vi "CfgLimitLines.vi"(0 "VISA IN":refnum<visa-resource-name>, 1 "Stimulus Start":dbl=1000000000.0, 2 "Stimulus Stop":dbl=2000000000.0, 3 "Amplitude Start":i32=-13, 4 "Amplitude Stop":i32=-14, 5 "Segment Limit":string(combo)="LMAX", 6 "Filename":string="CH1_S11_1", 7 "error in":errorcluster, 8 "Display Limit\n Segments ON/OFF":bool=TRUE, 9 "Channel":i32=1, 10 "Sound ON/OFF":bool=TRUE, 11 "Window":i32=1, 12 "Limit Testing ON/OFF":bool=TRUE, 13 "Segment number":i32=1, 14 "Show Table?":bool=TRUE) -> (20 "VISA Out":refnum<visa-resource-name>, 27 "error out":errorcluster)   [LabVIEW 2018, in "PNA-X.lvlib"]
uses:
  PNA-X.lvlib
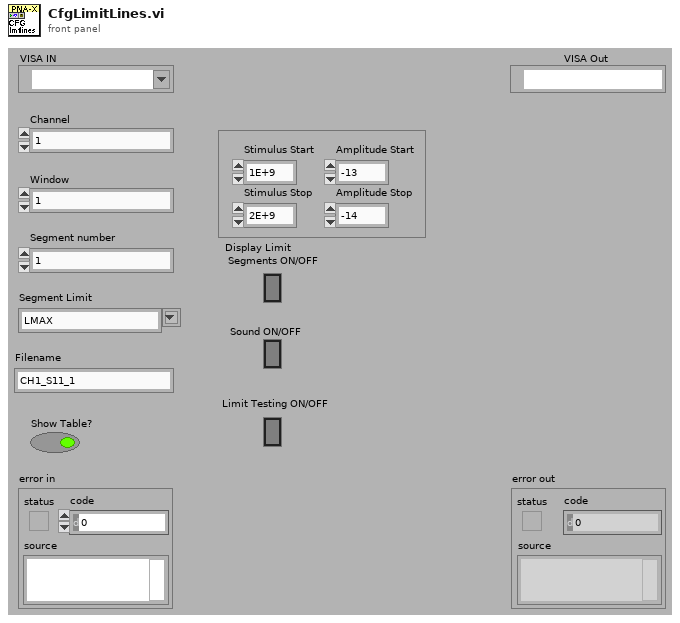
[diagram p1: front panel]
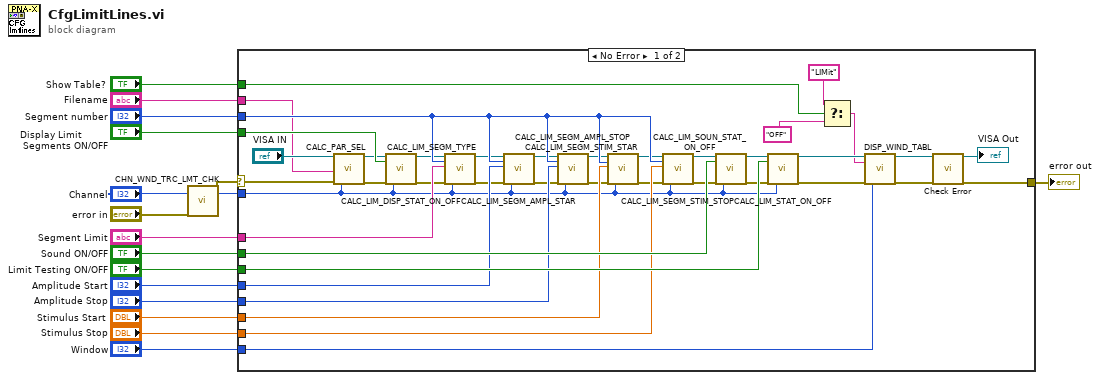
[diagram p0: block diagram]
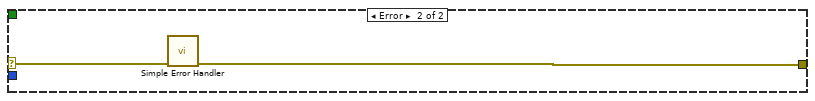
[diagram p2: hidden frame]
diagram:
  n1 = call "CHN_WND_TRC_LMT_CHK.vi"("Channel"="Channel", "error in"="error in") -> ("error out"=w4:errorcluster, "Channel"=w15:i32)  [unwired: 13 in, 3 out]
  n2 = case shown="No Error" w4 {
    selector: w4 -> [w44 w59]
    tunnel: [w57 w58] -> w16
    tunnel: w15 -> [w42 _]
    tunnel: "Display Limit\n Segments ON/OFF" -> [w55 _]
    tunnel: "Filename" -> [w41 _]
    tunnel: "Segment number" -> [w54 _]
    tunnel: "Sound ON/OFF" -> [w53 _]
    tunnel: "Limit Testing ON/OFF" -> [w52 _]
    tunnel: "Segment Limit" -> [w51 _]
    tunnel: "Amplitude Stop" -> [w50 _]
    tunnel: "Amplitude Start" -> [w49 _]
    tunnel: "Stimulus Start" -> [w48 _]
    tunnel: "Stimulus Stop" -> [w47 _]
    tunnel: "Window" -> [w22 _]
    tunnel: "Show Table?" -> [w21 _]
    frame No Error {
      n3 = call "CALC_PAR_SEL.vi"("VISA IN"="VISA IN", "Measurement"=w41, "error in"=w44, "Channel"=w42) -> ("VISA Out"=w45:refnum<visa-resource-name>, "error out"=w43:errorcluster)  [unwired: 14 in]
      n4 = call "CALC_LIM_DISP_STAT_ON_OFF.vi"("VISA IN"=w45, "Display Limit Segments ON/OFF"=w55, "error in"=w43, "Channel"=w42) -> ("VISA Out"=w40:refnum<visa-resource-name>, "error out"=w39:errorcluster)  [unwired: 14 in]
      n5 = call "CALC_LIM_SEGM_TYPE.vi"("VISA IN"=w40, "Segment number"=w54, "Segment Limit"=w51, "error in"=w39, "Channel"=w42) -> ("VISA Out"=w38:refnum<visa-resource-name>, "error out"=w37:errorcluster)  [unwired: 13 in]
      n6 = call "CALC_LIM_SEGM_AMPL_STAR.vi"("VISA IN"=w38, "Segment number"=w54, "Start number"=w49, "error in"=w37, "Channel"=w42) -> ("VISA Out"=w36:refnum<visa-resource-name>, "error out"=w35:errorcluster)  [unwired: 13 in]
      n7 = call "CALC_LIM_SEGM_AMPL_STOP.vi"("VISA IN"=w36, "Segment number"=w54, "Stop number"=w50, "error in"=w35, "Channel"=w42) -> ("VISA Out"=w34:refnum<visa-resource-name>, "error out"=w33:errorcluster)  [unwired: 13 in]
      n8 = call "CALC_LIM_SEGM_STIM_STAR.vi"("VISA IN"=w34, "Segment number"=w54, "Start number"=w48, "error in"=w33, "Channel"=w42) -> ("VISA Out"=w32:refnum<visa-resource-name>, "error out"=w31:errorcluster)  [unwired: 13 in]
      n9 = call "CALC_LIM_SEGM_STIM_STOP.vi"("VISA IN"=w32, "Segment number"=w54, "Stop number"=w47, "error in"=w31, "Channel"=w42) -> ("VISA Out"=w30:refnum<visa-resource-name>, "error out"=w29:errorcluster)  [unwired: 13 in]
      n10 = call "CALC_LIM_SOUN_STAT_ON_OFF.vi"("VISA IN"=w30, "Sound ON/OFF"=w53, "error in"=w29, "Channel"=w42) -> ("VISA Out"=w28:refnum<visa-resource-name>, "error out"=w27:errorcluster)  [unwired: 14 in]
      n11 = call "CALC_LIM_STAT_ON_OFF.vi"("VISA IN"=w28, "Limit Testing ON/OFF"=w52, "error in"=w27, "Channel"=w42) -> ("VISA Out"=w26:refnum<visa-resource-name>, "error out"=w25:errorcluster)  [unwired: 14 in]
      n12 = Select(t="LIMit" ("Tables"), s=w21, f="OFF" ("Tables")) -> (s? t:f=w18:string)
      n13 = call "DISP_WIND_TABL.vi"("VISA IN"=w26, "Tables"=w18, "error in"=w25, "Window"=w22) -> ("VISA Out"=w23:refnum<visa-resource-name>, "error out"=w24:errorcluster)  [unwired: 14 in]
      n14 = call "Check Error.vi"("VISA Resource Name"=w23, "error in (no error)"=w24) -> ("dup VISA session"=→"VISA Out":refnum<visa-resource-name>, "error out"=w57:errorcluster)  [unwired: 16 in]
    }
    frame Error {
      n15 = call <vilib>:"Simple Error Handler.vi"("error in (no error)"=w59) -> ("error out"=w58:errorcluster)  [unwired: 4 in, 4 out]
    }
  }
  "error out" <- w16
